vi "trig_level_ctrl.vi"(10 "std":dbl, 11 "mean":dbl) -> ()   [LabVIEW 2019]
panel:
  in  "trig1 level":dbl(slide)=783.9195979899498 scale=0.0..2000.0
  out "Tank":dbl(slide) scale=0.0..2000.0
  out "Tank 4":dbl(slide) scale=0.0..2000.0
  out "Tank 3":dbl(slide) scale=0.0..2000.0
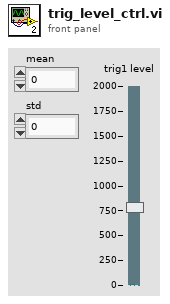
[diagram p1: front panel]
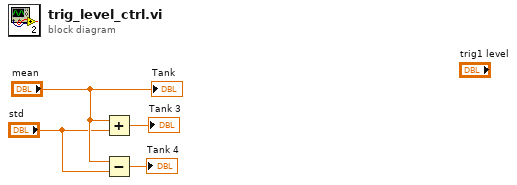
[diagram p0: block diagram]
diagram:
  n1 = Add(x="mean", y="std") -> (x+y=→"Tank 3":dbl)
  n2 = Subtract(x="mean", y="std") -> (x-y=→"Tank 4":dbl)
  "Tank" <- "mean"
